vi "Read Measurement Result (Single Point).vi"(7 "Maximum Time (10000 ms)":i32=10000, 8 "error in (no error)":errorcluster, 9 "Data Mode (5: Voltage)":i32(ring)=5 items=["Current", "Resistance", "Source Output Setting", "Status", "Time", "Voltage"], 10 "Channel (0: Channel 1)":i32(ring) items=["Channel 1", "Channel 2"], 11 "VISA resource name":refnum<visa-resource-name>) -> (0 "error out":errorcluster, 2 "Measurement Result":dbl, 3 "VISA resource name out":refnum<visa-resource-name>)   [LabVIEW 2023, in "Agilent B2900 Series.lvlib"]
doc: "Reads and fetch the latest data in series."
uses:
  Agilent B2900 Series.lvlib
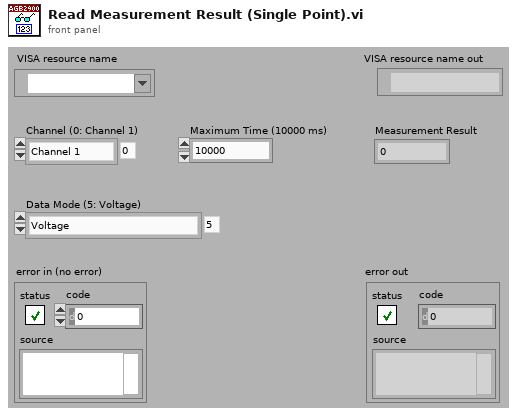
[diagram p1: front panel]
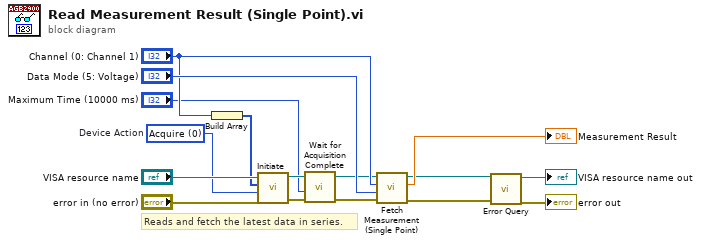
[diagram p0: block diagram]
diagram:
  w11 = 0 items=["Acquire", "Transient", "Both"]  # Device Action
  # "Reads and fetch the latest data in series."
  n1 = Build Array("Channel (0: Channel 1)") -> (w12:i32[])
  n2 = call "Initiate.vi"("error in (no error)"="error in (no error)", "Device Action (2: Both)"=w11, "Channel List ({Channel1})"=w12, "VISA resource name"="VISA resource name") -> ("error out"=w4:errorcluster, "VISA resource name out"=w5:refnum<visa-resource-name>)  [unwired: 6 in]
  n3 = call "Wait for Acquisition Complete.vi"("error in (no error)"=w4, "Maximum Time (10000 ms)"="Maximum Time (10000 ms)", "VISA resource name"=w5) -> ("error out"=w2:errorcluster, "VISA resource name out"=w3:refnum<visa-resource-name>)  [unwired: 7 in]
  n4 = call "Fetch Measurement (Single Point).vi"("error in (no error)"=w2, "Data Mode (5: Voltage)"="Data Mode (5: Voltage)", "Channel (0: Channel 1)"="Channel (0: Channel 1)", "VISA resource name"=w3) -> ("error out"=w6:errorcluster, "Measurement"=→"Measurement Result":dbl, "VISA resource name out"=w7:refnum<visa-resource-name>)  [unwired: 5 in]
  n5 = call "Error Query.vi"("error in (no error)"=w6, "VISA resource name"=w7) -> ("error out"=→"error out":errorcluster, "VISA resource name out"=→"VISA resource name out":refnum<visa-resource-name>)  [unwired: 6 in, 2 out]
